vi "密码修改.vi"() -> ()   [LabVIEW 2015]
panel:
  in  "确定修改":bool
  in  "新密码：":string
  in  "新账户：":string
  in  "密码：":string
  in  "账户：":string
  in  "原密码所在位置":path=path "E:/桌面/Desktop/登录测试/user.txt"
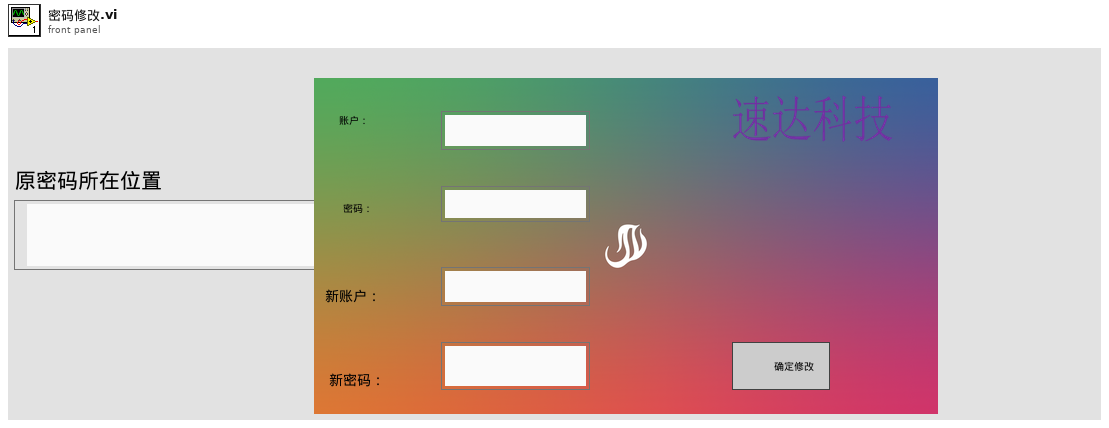
[diagram p1: front panel]
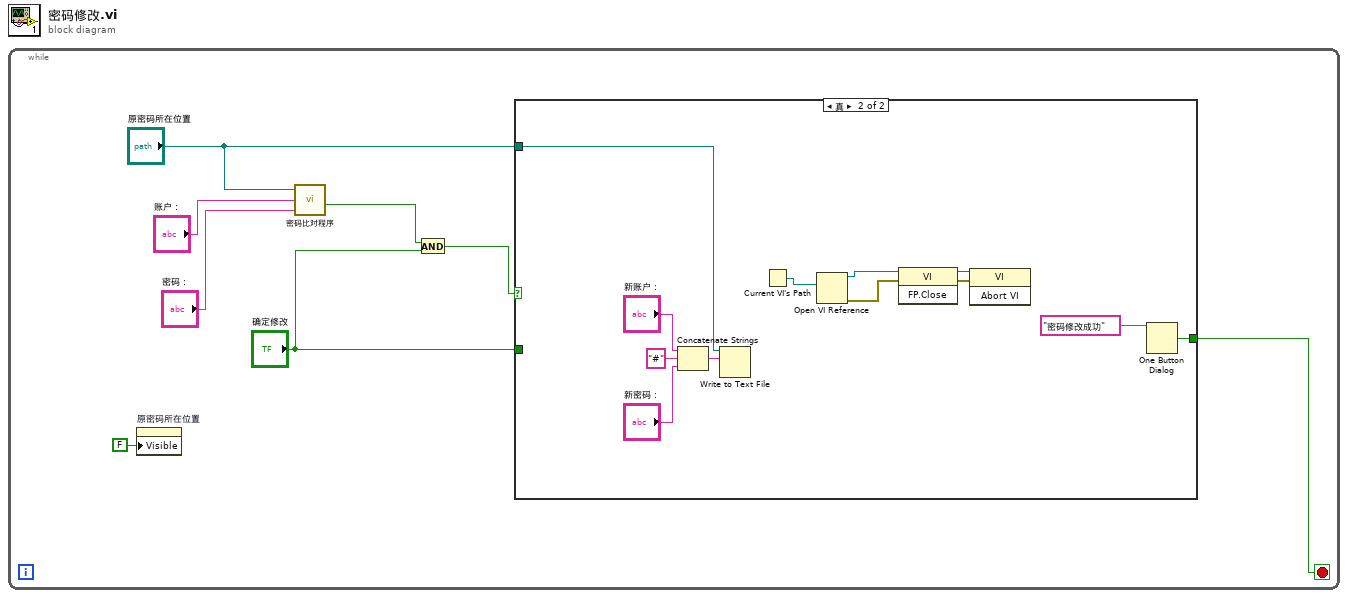
[diagram p0: block diagram]
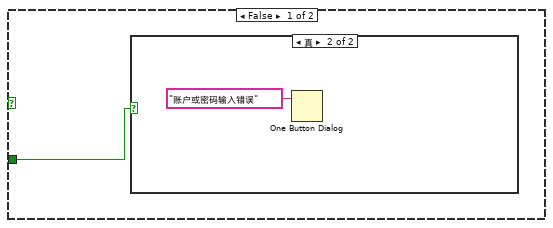
[diagram p2: hidden frame]
diagram:
  n1 = while {
    stop <- w2 stop-if-true
    n2 = property on="原密码所在位置" class="Path"("Visible"=FALSE ("可见")) -> ()  [unwired: 2 in, 2 out]
    n3 = call "密码比对程序.vi"("密码"="密码：", "账户"="账户：", "原密码所在位置"="原密码所在位置") -> ("x = y?"=w6:bool)  [unwired: 5 in]
    n4 = And(x=w6, y="确定修改") -> (x .and. y?=w5:bool)
    n5 = case shown="真" w5 {
      tunnel: "原密码所在位置" -> [_ w18]
      tunnel: "确定修改" -> [w9 _]
      tunnel: [_ w11] -> w2
      frame False {
        n6 = case shown="真" w9 {
          frame False {
          }
          frame True {
            n7 = One Button Dialog(message="账户或密码输入错误" ("消息")) -> ()  [unwired: 1 in, 1 out]
          }
        }
      }
      frame True {
        n8 = Concatenate Strings("新账户：", "#" ("字符串"), "新密码：") -> (w19:string)
        n9 = Write to Text File(file (use dialog)=w18, text=w19) -> ()  [unwired: 2 in, 3 out]
        n10 = Current VI's Path() -> (path=w14:path)
        n11 = Open VI Reference(vi path=w14) -> (vi reference=w16:refnum<vi>, error out=w15:errorcluster)  [unwired: 5 in]
        n12 = invoke class="VI" method="FP.Close"(reference=w16, error in=w15) -> (reference out=w13:refnum<vi>, error out=w12:errorcluster)  [unwired: 1 in, 1 out]
        n13 = invoke class="VI" method="Abort VI"(reference=w13, error in=w12) -> ()  [unwired: 1 in, 3 out]
        n14 = One Button Dialog(message="密码修改成功" ("消息")) -> (true=w11:bool)  [unwired: 1 in]
      }
    }
  }
